vi "Initialize CAN.vi"(8 "error in (no error)":errorcluster, 11 "Parameters":T1={"Properties"={"Name"="", "CAN"={"Database File"=path "", "CAN Interface"=enum."CAN0", "Baud Rate"=0, "Diagnostic Protocol"=enum."GMLAN", "Transport Protocol"=enum."ISO TP - Normal Mode", "Transmit ID"=0, "Receive ID"=0, "Transmit Extension"=0, "Receive Extension"=0, "Receive UUDT ID"=0, "Enable Stream"=TRUE, "VW TP Channel ID"=0, "Security"={"Source DLL Path"=path "", "Security Level"=1, "Target DLL Path"=path ""}, "Fill Frame"=FALSE, "Fill Byte"=255, "Termination"=FALSE}, "FPGA Settings"={"RT Bitfile Path"=path "", "RIO Device"=0, "Enable"=FALSE}, "PIDs"=[], "PID Lookup"=variant, "CPIDs"=[], "CPID Lookup"=variant, "DIDs"=[], "DID Lookup"=variant, "DPIDs"=[], "DPID Lookup"=variant, "DTC descriptor"={"DTC Byte Length"=2, "Status Byte Length"=1, "Add Data Byte Length"=1, "Byte Order"=enum."Motorola"}}, "ChanRefs"={"ToVS.PIDs"={"Name"="", "Write to VS Engine FIFO"=refnum, "Pairs"={"Refs"=[], "Values"=[]}}, "ToVS.DIDs"={"Name"="", "Write to VS Engine FIFO"=refnum, "Pairs"={"Refs"=[], "Values"=[]}}, "ToVS.DTCs"={"Name"="", "Write to VS Engine FIFO"=refnum, "Pairs"={"Refs"=[], "Values"=[]}}, "ToVS.DTCCount"={"Name"="", "Write to VS Engine FIFO"=refnum, "Pairs"={"Refs"=[], "Values"=[]}}, "ToVS.Success"={"Name"="", "Write to VS Engine FIFO"=refnum, "Pairs"={"Refs"=[], "Values"=[]}}, "FromVS.CPIDs"={"Name"="", "Read from VS Engine FIFO"=refnum, "Pairs"={"Refs"=[], "Values"=[]}}, "Cmds"={"Name"="", "Write to VS Engine FIFO"=refnum, "Read from VS Engine FIFO"=refnum, "Pairs"={"Chan Refs"=[], "Prev. Values"=[]}}}} {"ChanRefs"."Cmds"."Pairs"."Chan Refs" format="%.0x"; "ChanRefs"."FromVS.CPIDs"."Pairs"."Refs"."Data Reference" format="%.0x"; "ChanRefs"."ToVS.Success"."Pairs"."Refs" format="%.0x"; "ChanRefs"."ToVS.DTCCount"."Pairs"."Refs" format="%.0x"; "ChanRefs"."ToVS.DTCs"."Pairs"."Refs" format="%.0x"; "ChanRefs"."ToVS.PIDs"."Pairs"."Refs" format="%.0x"; "ChanRefs"."ToVS.DIDs"."Pairs"."Refs" format="%.0x"; "Properties"."CPIDs"."Signals"."Byte Order" items=["Little Endian", "Big Endian"]; "Properties"."CPIDs"."Signals"."Data Type" items=["Signed", "Unsigned", "IEEE Float"]; "Properties"."DIDs"."Signals"."Byte Order" items=["Little Endian", "Big Endian"]; "Properties"."DIDs"."Signals"."Data Type" items=["Signed", "Unsigned", "IEEE Float"]; "Properties"."CAN"."Fill Byte" format="%.0x"; "Properties"."CAN"."VW TP Channel ID" format="%.0x"; "Properties"."CAN"."Receive UUDT ID" format="%.0x"; "Properties"."CAN"."Receive Extension" format="%.0x"; "Properties"."CAN"."Transmit Extension" format="%.0x"; "Properties"."CAN"."Receive ID" format="%.0x"; "Properties"."CAN"."Transmit ID" format="%.0x"; "Properties"."PIDs"."Signals"."Byte Order" items=["Little Endian", "Big Endian"]; "Properties"."PIDs"."Signals"."Data Type" items=["Signed", "Unsigned", "IEEE Float"]}) -> (0 "error out":errorcluster, 1 "ADCS Connection":T21, 2 "XNET References":T20, 3 "Parameters":T1={"Properties"={"Name"="", "CAN"={"Database File"=path "", "CAN Interface"=enum."CAN0", "Baud Rate"=0, "Diagnostic Protocol"=enum."GMLAN", "Transport Protocol"=enum."ISO TP - Normal Mode", "Transmit ID"=0, "Receive ID"=0, "Transmit Extension"=0, "Receive Extension"=0, "Receive UUDT ID"=0, "Enable Stream"=TRUE, "VW TP Channel ID"=0, "Security"={"Source DLL Path"=path "", "Security Level"=1, "Target DLL Path"=path ""}, "Fill Frame"=FALSE, "Fill Byte"=255, "Termination"=FALSE}, "FPGA Settings"={"RT Bitfile Path"=path "", "RIO Device"=0, "Enable"=FALSE}, "PIDs"=[], "PID Lookup"=variant, "CPIDs"=[], "CPID Lookup"=variant, "DIDs"=[], "DID Lookup"=variant, "DPIDs"=[], "DPID Lookup"=variant, "DTC descriptor"={"DTC Byte Length"=2, "Status Byte Length"=1, "Add Data Byte Length"=1, "Byte Order"=enum."Motorola"}}, "ChanRefs"={"ToVS.PIDs"={"Name"="", "Write to VS Engine FIFO"=refnum, "Pairs"={"Refs"=[], "Values"=[]}}, "ToVS.DIDs"={"Name"="", "Write to VS Engine FIFO"=refnum, "Pairs"={"Refs"=[], "Values"=[]}}, "ToVS.DTCs"={"Name"="", "Write to VS Engine FIFO"=refnum, "Pairs"={"Refs"=[], "Values"=[]}}, "ToVS.DTCCount"={"Name"="", "Write to VS Engine FIFO"=refnum, "Pairs"={"Refs"=[], "Values"=[]}}, "ToVS.Success"={"Name"="", "Write to VS Engine FIFO"=refnum, "Pairs"={"Refs"=[], "Values"=[]}}, "FromVS.CPIDs"={"Name"="", "Read from VS Engine FIFO"=refnum, "Pairs"={"Refs"=[], "Values"=[]}}, "Cmds"={"Name"="", "Write to VS Engine FIFO"=refnum, "Read from VS Engine FIFO"=refnum, "Pairs"={"Chan Refs"=[], "Prev. Values"=[]}}}} {"ChanRefs"."Cmds"."Pairs"."Chan Refs" format="%.0x"; "ChanRefs"."FromVS.CPIDs"."Pairs"."Refs"."Data Reference" format="%.0x"; "ChanRefs"."ToVS.Success"."Pairs"."Refs" format="%.0x"; "ChanRefs"."ToVS.DTCCount"."Pairs"."Refs" format="%.0x"; "ChanRefs"."ToVS.DTCs"."Pairs"."Refs" format="%.0x"; "ChanRefs"."ToVS.PIDs"."Pairs"."Refs" format="%.0x"; "ChanRefs"."ToVS.DIDs"."Pairs"."Refs" format="%.0x"; "Properties"."CPIDs"."Signals"."Byte Order" items=["Little Endian", "Big Endian"]; "Properties"."CPIDs"."Signals"."Data Type" items=["Signed", "Unsigned", "IEEE Float"]; "Properties"."DIDs"."Signals"."Byte Order" items=["Little Endian", "Big Endian"]; "Properties"."DIDs"."Signals"."Data Type" items=["Signed", "Unsigned", "IEEE Float"]; "Properties"."CAN"."Fill Byte" format="%.0x"; "Properties"."CAN"."VW TP Channel ID" format="%.0x"; "Properties"."CAN"."Receive UUDT ID" format="%.0x"; "Properties"."CAN"."Receive Extension" format="%.0x"; "Properties"."CAN"."Transmit Extension" format="%.0x"; "Properties"."CAN"."Receive ID" format="%.0x"; "Properties"."CAN"."Transmit ID" format="%.0x"; "Properties"."PIDs"."Signals"."Byte Order" items=["Little Endian", "Big Endian"]; "Properties"."PIDs"."Signals"."Data Type" items=["Signed", "Unsigned", "IEEE Float"]})   [LabVIEW 2015, in "Diagnostics Addon Engine.lvlib"]
uses:
  Diagnostics Addon Engine.lvlib
  Main Configuration.ctl
  Shared/Section Properties.ctl
  Shared/CAN Configuration.ctl
  Shared/CAN Interface.ctl
  Shared/Diagnostic Protocols.ctl
  Shared/Transport Protocols.ctl
  Shared/Security.ctl
  Shared/FPGA Bitfile Settings.ctl
  Shared/Frame Parameters.ctl
  Shared/Signal Parameters.ctl
  Shared/DPID Parameters.ctl
  Shared/DPID Periodic Rate.ctl
  <vilib>/Automotive Diagnostic Command Set/Diagnostic Protocols.llb/DTC Descriptor.ctl
  VS Data Channels.ctl
  Inline Async API/Controls/Write To VS Engine.ctl
  <vilib>/NI Veristand/Custom Device API/Data Reference.ctl
  Inline Async API/Controls/Read From VS Engine.ctl
  <vilib>/NI Veristand/Custom Device API/Block Data Reference.ctl
  Inline Async API/Controls/ReadWrite Data.ctl
  <vilib>/Automotive Diagnostic Command Set/Diagnostic Transport.llb/Diag Reference.ctl
  <vilib>/Automotive Diagnostic Command Set/Diagnostic Transport.llb/Transport Protocol Selector.ctl
  <vilib>/Automotive Diagnostic Command Set/Diagnostic Transport.llb/Diag CAN Frame Log.ctl
  XNET References.ctl
  <vilib>/Automotive Diagnostic Command Set/Diagnostic Transport.llb/Property ID.ctl
  DIDPID Selector.ctl
  <vilib>/Automotive Diagnostic Command Set/Diagnostic Transport.llb/VWTP Application Type.ctl
  <vilib>/Automotive Diagnostic Command Set/Diagnostic Transport.llb/DoIP OpenType.ctl
  <vilib>/xnet/xnet.llb/XNET Create Session (Frame Input Queued).vi
  <vilib>/addons/Automotive Diagnostic Command Set/NI_Automotive Diagnostic Command Set.lvlib
  <vilib>/NI Veristand/Custom Device Tools/Custom Device Utility Library/Custom Device Utility Library.lvlib
  Shared/Diagnostics Addon Shared.lvlib
  <vilib>/NI Veristand/Custom Device API/Custom Device API.lvlib
  Inline Async API/Inline Async API.lvlib
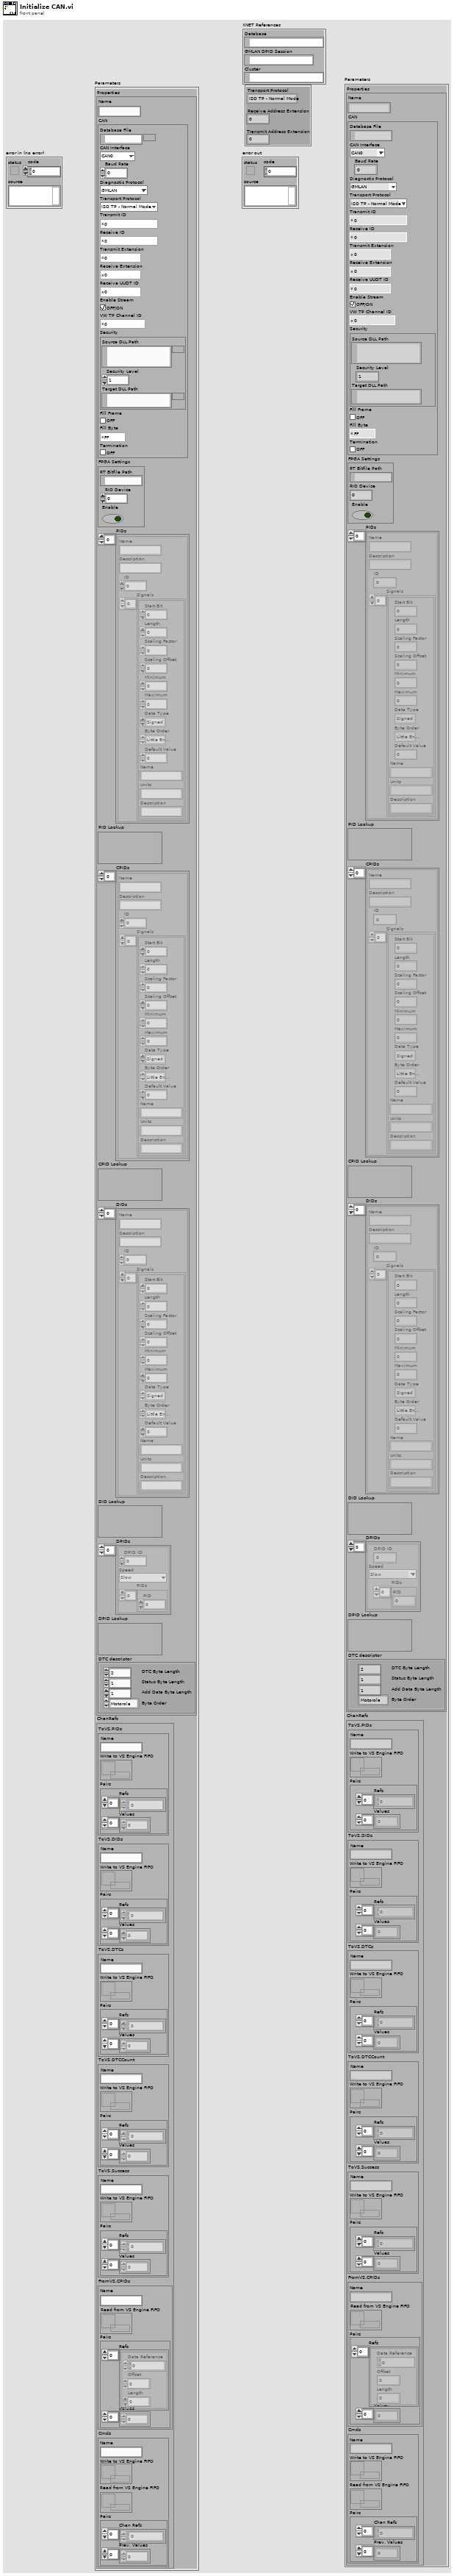
[diagram p1: front panel]
types:
  T1 = typedef "Diagnostics Addon Engine.lvlib/Main Configuration.ctl" = cluster{"Properties":T2, "ChanRefs":T14}
  T2 = typedef "Diagnostics Addon Shared.lvlib/Section Properties.ctl" = cluster{"Name":string, "CAN":T3, "FPGA Settings":T8, "PIDs":T9[], "PID Lookup":variant, "CPIDs":T9[], "CPID Lookup":variant, "DIDs":T9[], "DID Lookup":variant, "DPIDs":T11[], "DPID Lookup":variant, "DTC descriptor":T13}
  T3 = typedef "Diagnostics Addon Shared.lvlib/CAN Configuration.ctl" = cluster{"Database File":path, "CAN Interface":T4, "Baud Rate":u32, "Diagnostic Protocol":T5, "Transport Protocol":T6, "Transmit ID":u32, "Receive ID":u32, "Transmit Extension":u8, "Receive Extension":u8, "Receive UUDT ID":u32, "Enable Stream":bool, "VW TP Channel ID":u32, "Security":T7, "Fill Frame":bool, "Fill Byte":u8, "Termination":bool}
  T4 = typedef "Diagnostics Addon Shared.lvlib/CAN Interface.ctl" = enum16{"CAN0", "CAN1", "CAN2", "CAN3", "CAN4", "CAN5", "CAN6", "CAN7", "CAN8", "CAN9", "CAN10", "CAN11", "CAN12", "CAN13", "CAN14", "CAN15", "CAN16", "CAN17", "CAN18", "CAN19", "CAN20", "CAN21", "CAN22", "CAN23", "CAN24", "CAN25", "CAN26", "CAN27", "CAN28", "CAN29", "CAN30", "CAN31", "CAN32", "CAN33", "CAN34", "CAN35", "CAN36", "CAN37", "CAN38", "CAN39", "CAN40", "CAN41", "CAN42", "CAN43", "CAN44", "CAN45", "CAN46", "CAN47", "CAN48", "CAN49", "CAN50", "CAN51", "CAN52", "CAN53", "CAN54", "CAN55", "CAN56", "CAN57", "CAN58", "CAN59", "CAN60", "CAN61", "CAN62", "CAN63", "CAN 256 (Virtual)", "CAN 257 (Virtual)"}
  T5 = typedef "Diagnostics Addon Shared.lvlib/Diagnostic Protocols.ctl" = enum16{"GMLAN", "KWP-2000", "UDS"}
  T6 = typedef "Diagnostics Addon Shared.lvlib/Transport Protocols.ctl" = enum16{"ISO TP - Normal Mode", "ISO TP - Mixed Mode", "VW TP 2.0", "Diagnostics on IP"}
  T7 = typedef "Diagnostics Addon Shared.lvlib/Security.ctl" = cluster{"Source DLL Path":path, "Security Level":u8, "Target DLL Path":path}
  T8 = typedef "Diagnostics Addon Shared.lvlib/FPGA Bitfile Settings.ctl" = cluster{"RT Bitfile Path":path, "RIO Device":u16, "Enable":bool}
  T9 = typedef "Diagnostics Addon Shared.lvlib/Frame Parameters.ctl" = cluster{"Name":string, "Description":string, "ID":u16, "Signals":T10[]}
  T10 = typedef "Diagnostics Addon Shared.lvlib/Signal Parameters.ctl" = cluster{"Start Bit":u8, "Length":u8, "Scaling Factor":dbl, "Scaling Offset":dbl, "Minimum":dbl, "Maximum":dbl, "Data Type":u32, "Byte Order":u32, "Default Value":dbl, "Name":string, "Units":string, "Description":string}
  T11 = typedef "Diagnostics Addon Shared.lvlib/DPID Parameters.ctl" = cluster{"DPID ID":u8, "Speed":T12, "PIDs":u16[]}
  T12 = typedef "Diagnostics Addon Shared.lvlib/DPID Periodic Rate.ctl" = enum16{"Slow", "Medium", "Fast"}
  T13 = typedef "Diagnostics Addon Shared.lvlib/DTC Descriptor.ctl" = cluster{"DTC Byte Length":i32, "Status Byte Length":i32, "Add Data Byte Length":i32, "Byte Order":enum16{"Motorola", "Intel"}}
  T14 = typedef "Diagnostics Addon Engine.lvlib/VS Data Channels.ctl" = cluster{"ToVS.PIDs":T15, "ToVS.DIDs":T15, "ToVS.DTCs":T15, "ToVS.DTCCount":T15, "ToVS.Success":T15, "FromVS.CPIDs":T17, "Cmds":T19}
  T15 = typedef "Diagnostics Addon Engine.lvlib/Inline Async API.lvlib/Write To VS Engine.ctl" = cluster{"Name":string, "Write to VS Engine FIFO":refnum<k33>, "Pairs":cluster{"Refs":T16[], "Values":dbl[]}}
  T16 = typedef "Custom Device API.lvlib/Data Reference.ctl" = i32
  T17 = typedef "Diagnostics Addon Engine.lvlib/Inline Async API.lvlib/Read From VS Engine.ctl" = cluster{"Name":string, "Read from VS Engine FIFO":refnum<k33>, "Pairs":cluster{"Refs":T18[], "Values":dbl[]}}
  T18 = typedef "Custom Device API.lvlib/Block Data Reference.ctl" = cluster{"Data Reference":T16, "Offset":u64, "Length":u64}
  T19 = typedef "Diagnostics Addon Engine.lvlib/Inline Async API.lvlib/ReadWrite Data.ctl" = cluster{"Name":string, "Write to VS Engine FIFO":refnum<k33>, "Read from VS Engine FIFO":refnum<k33>, "Pairs":cluster{"Chan Refs":T16[], "Prev. Values":dbl[]}}
  T20 = typedef "Diagnostics Addon Engine.lvlib/XNET References.ctl" = cluster{"Database":refnum<k21>, "GMLAN DPID Session":refnum<k21>, "Cluster":refnum<k21>}
  T21 = typedef "NI_Automotive Diagnostic Command Set.lvlib/Diag Reference.ctl" = cluster{"Diag CAN Handle":u32, "Transport Protocol":T22, "Receive Address Extension":u8, "Transmit Address Extension":u8, "Receive CAN Id":u32, "Transmit CAN Id":u32, "Diag CAN Queue":refnum<queue>, "Log Frames ?":bool, "My TP Address":u8, "Other TP Address":u8, "T1":u16, "T2":u16, "T3":u16, "T4":u16, "Tx SN":u8, "Block Size":u8, "Rx SN":u8, "VW TP Initialized?":bool, "Tx block no":u8, "baud rate":u32, "Interface":string, "Channel Diag CAN Handle":u32, "UDP Connection ID":refnum<k16>, "TCP Connection ID":refnum<k5>, "Target IP Addr":u32, "Source Address":u16, "Target Address":u16, "Send Header NACK?":bool, "DLL Handle":u32, "NAD":u8, "Time Stamp read first":dbl, "Time Stamp read last":dbl, "Time Stamp write first":dbl, "Time Stamp write last":dbl, "Time Stamp write":dbl, "Time Stamp read":dbl}
  T22 = typedef "NI_Automotive Diagnostic Command Set.lvlib/Transport Protocol Selector.ctl" = enum16{"ISO TP - Normal Mode", "ISO TP - Mixed Mode", "VW TP 2.0", "Diagnostics on IP", "ISO TP LIN"}
  T23 = typedef "NI_Automotive Diagnostic Command Set.lvlib/Property ID.ctl" = enum16{"Timeout Diag Command", "Timeout FC (Bs)", "Timeout CF (Cr)", "Receive Block Size (BS)", "Wait Time CF (STmin)", "Max Wait Frames (N_WFTmax)", "Wait Frames to Send (N_WAIT)", "Time between Waits (T_W)", "Fill CAN Frames", "Fill Byte", "Invalid Response as Error", "Max RspPending Count", "VWTP Command Timeout", "STmin", "P2min", "Termination"}
  T24 = typedef "Diagnostics Addon Engine.lvlib/DIDPID Selector.ctl" = enum16{"DID", "PID", "CPID"}
  T25 = typedef "NI_Automotive Diagnostic Command Set.lvlib/VWTP Application Type.ctl" = u8
  T26 = typedef "NI_Automotive Diagnostic Command Set.lvlib/DoIP OpenType.ctl" = u16
  T27 = typedef "NI_Automotive Diagnostic Command Set.lvlib/DoIP Vehicle ID Cluster.ctl" = cluster{"VIN":string, "Source Address":u16, "EID":u8[], "GID":u8[], "IP Address":string}
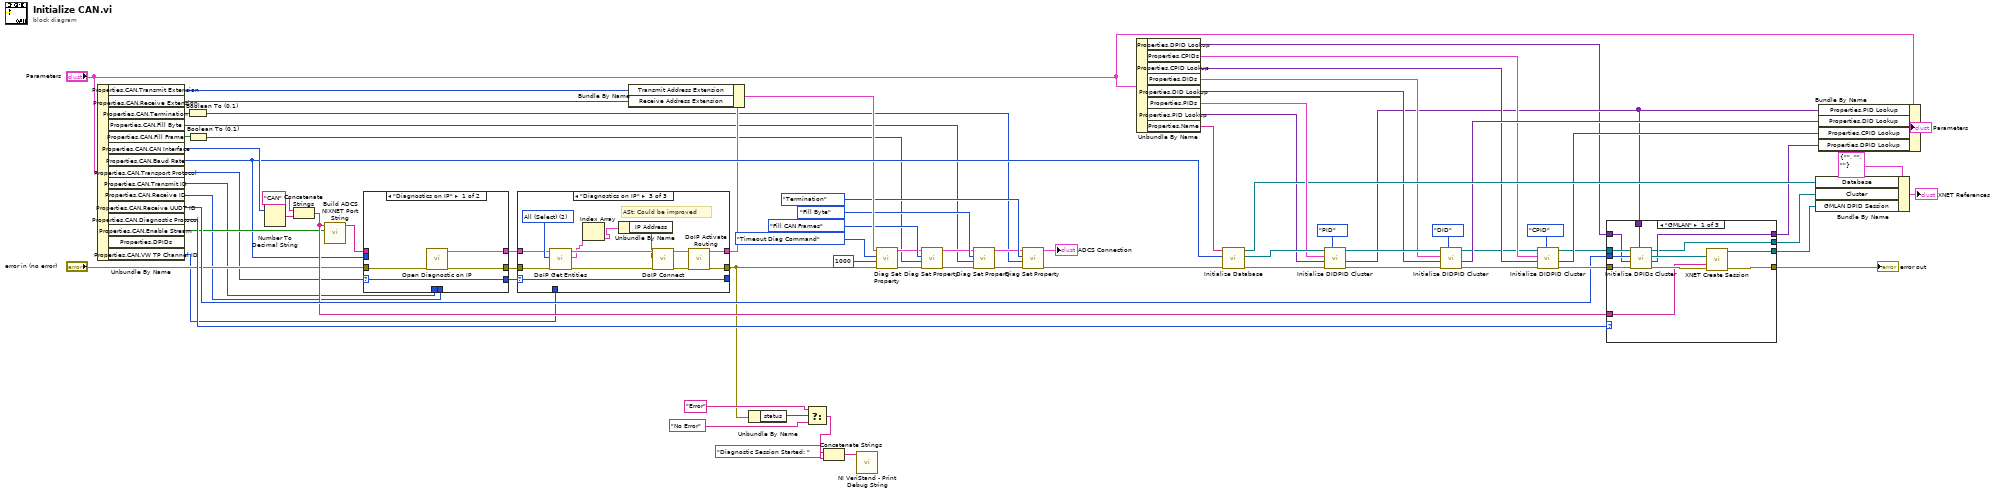
[diagram p0: block diagram]
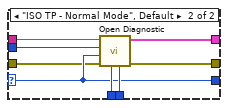
[diagram p2: hidden frame]
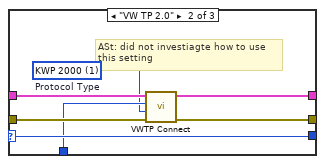
[diagram p4: hidden frame]
diagram:
  n1 = Unbundle By Name("Parameters") -> ("Properties.CAN.Transmit Extension"=w74:u8, "Properties.CAN.Receive Extension"=w73:u8, "Properties.CAN.Termination"=w3:bool, "Properties.CAN.Fill Byte"=w5:u8, "Properties.CAN.Fill Frame"=w4:bool, "Properties.CAN.CAN Interface"=w77:T4, "Properties.CAN.Baud Rate"=w25:u32, "Properties.CAN.Transport Protocol"=w28:T6, "Properties.CAN.Transmit ID"=w24:u32, "Properties.CAN.Receive ID"=w23:u32, "Properties.CAN.Receive UUDT ID"=w44:u32, "Properties.CAN.Diagnostic Protocol"=w43:T5, "Properties.CAN.Enable Stream"=w37:bool, "Properties.CAN.VW TP Channel ID"=w18:u32)  [unwired: 1 out]
  n2 = Boolean To (0,1)(Boolean=w3) -> (0, 1=w2:i16)
  n3 = Boolean To (0,1)(Boolean=w4) -> (0, 1=w1:i16)
  n4 = Number To Decimal String(number=w77) -> (decimal integer string=w76:string)  [unwired: 1 in]
  n5 = Concatenate Strings("CAN" ("string"), w76) -> (w38:string)
  n6 = call "Build ADCS NIXNET Port String.vi"("Enable Stream"=w37, "CAN port"=w38) -> ("CAN port out"=w26:string)  [unwired: 9 in]
  n7 = case shown="\"Diagnostics on IP\"" w28 {
    selector: w28 -> [w81 w83]
    tunnel: w24 -> [_ w89]
    tunnel: w25 -> [_ w88]
    tunnel: w23 -> [_ w87]
    tunnel: [w79 w86] -> w22
    tunnel: [w80 w85] -> w20
    tunnel: w26 -> [_ w84]
    tunnel: [w81 w83] -> w27
    tunnel: "error in (no error)" -> [w78 w82]
    frame "Diagnostics on IP" {
      n8 = call <vilib>:"Open Diagnostic on IP.vi"("error in (no error)"=w78) -> ("error out"=w80:errorcluster, "Diag reference out"=w79:T21)  [unwired: 1 in, 8 out]
    }
    frame "ISO TP - Normal Mode", Default {
      n9 = call <vilib>:"Open Diagnostic.vi"("Receive ID"=w87, "Transmit ID"=w89, "error in (no error)"=w82, "Transport Protocol"=w83, "Baud Rate"=w88, "CAN Interface"=w84) -> ("error out"=w85:errorcluster, "diag ref out"=w86:T21)  [unwired: 4 out]
    }
  }
  n10 = case shown="\"Diagnostics on IP\"" w27 {
    selector: w27 -> [w92 w97 w102]
    tunnel: [w91 w99 w105] -> w21
    tunnel: [w90 w98 w103] -> w19
    tunnel: [w92 w97 w102] -> _
    tunnel: w22 -> [w91 w96 w101]
    tunnel: w20 -> [w90 w95 w100]
    tunnel: w18 -> [_ w94 _]
    frame "ISO TP - Normal Mode", Default {
    }
    frame "VW TP 2.0" {
      w93 = T25 1 items=["KWP 2000"=1, "KS Type 010C"=2, "Infotainment communication"=16, "Application protocol"=32, "WFS/WIV"=33]  # Protocol Type
      # "ASt: did not investiagte how to use\nthis setting"
      n11 = call <vilib>:"VWTP Connect.vi"("error in"=w95, "application type"=w93, "channel ID"=w94, "diag ref in"=w96) -> ("error out"=w98:errorcluster, "diag ref out"=w99:T21)  [unwired: 6 out]
    }
    frame "Diagnostics on IP" {
      w112 = T26 2 items=["VIN", "EID", "All (Select)"] ("DoIP Open Type")
      # "ASt: Could be improved"
      n12 = call <vilib>:"DoIP Get Entities.vi"("error in (no error)"=w100, "DoIP Open Type"=w112, "Diag reference in"=w101) -> ("error out"=w109:errorcluster, "DoIP entities"=w108:T27[], "Diag reference out"=w110:T21)  [unwired: 1 in, 5 out]
      n13 = Index Array(array=w108) -> (element=w107:T27)  [unwired: 1 in]
      n14 = Unbundle By Name(w107) -> ("IP Address"=w106:string)
      n15 = call <vilib>:"DoIP Connect.vi"("error in (no error)"=w109, "address"=w106, "Diag Reference in"=w110) -> ("error out"=w104:errorcluster, "Diag reference out"=w111:T21)  [unwired: 2 in, 5 out]
      n16 = call <vilib>:"DoIP Activate Routing.vi"("error in (no error)"=w104, "Diag reference in"=w111) -> ("error out"=w103:errorcluster, "Diag reference out"=w105:T21)  [unwired: 2 in, 6 out]
    }
  }
  n17 = Bundle By Name(cluster=w21, "Transmit Address Extension"=w74, "Receive Address Extension"=w73) -> (w17:T21)
  n18 = Unbundle By Name(w19) -> ("status"=w34:bool)
  n19 = Select(t="Error" ("string"), s=w34, f="No Error" ("string")) -> (s? t:f=w31:string)
  n20 = Concatenate Strings("Diagnostic Session Started: " ("string"), w31) -> (w30:string)
  n21 = call <vilib>:"NI VeriStand - Print Debug String.vi"("Message"=w30) -> ()  [unwired: 10 in, 1 out]
  n22 = call <vilib>:"Diag Set Property.vi"("error in (no error)"=w19, "property value"=u32 1000, "property ID"=Property_ID."Timeout Diag Command", "diag ref in"=w17) -> ("error out"=w14:errorcluster, "diag ref out"=w9:T21)  [unwired: 6 in]
  n23 = call <vilib>:"Diag Set Property.vi"("error in (no error)"=w14, "property value"=w1, "property ID"=Property_ID."Fill CAN Frames", "diag ref in"=w9) -> ("error out"=w16:errorcluster, "diag ref out"=w8:T21)  [unwired: 6 in]
  n24 = call <vilib>:"Diag Set Property.vi"("error in (no error)"=w16, "property value"=w5, "property ID"=Property_ID."Fill Byte", "diag ref in"=w8) -> ("error out"=w15:errorcluster, "diag ref out"=w7:T21)  [unwired: 6 in]
  n25 = call <vilib>:"Diag Set Property.vi"("error in (no error)"=w15, "property value"=w2, "property ID"=Property_ID."Termination", "diag ref in"=w7) -> ("error out"=w13:errorcluster, "diag ref out"=→"ADCS Connection":T21)  [unwired: 6 in]
  n26 = Unbundle By Name("Parameters") -> ("Properties.DPID Lookup"=w40:variant, "Properties.CPIDs"=w50:T9[], "Properties.CPID Lookup"=w51:variant, "Properties.DIDs"=w58:T9[], "Properties.DID Lookup"=w55:variant, "Properties.PIDs"=w60:T9[], "Properties.PID Lookup"=w56:variant, "Properties.Name"=w57:string)
  n27 = call "Initialize Database.vi"("error in (no error)"=w13, "Baud Rate"=w25, "Addon Name"=w57) -> ("error out"=w67:errorcluster, "Cluster"=w65:refnum<k21>, "XNET Database"=w59:refnum<k21>)  [unwired: 6 in]
  n28 = call "Initialize DIDPID Cluster.vi"("DID/PID Selector"=DIDPID_Selector."PID", "error in"=w67, "Lookup"=w56, "DIDs/PIDs"=w60, "Cluster In"=w65) -> ("error out"=w66:errorcluster, "DID Lookup Out"=w41:variant, "Cluster Out"=w62:refnum<k21>)  [unwired: 4 in]
  n29 = call "Initialize DIDPID Cluster.vi"("DID/PID Selector"=DIDPID_Selector."DID", "error in"=w66, "Lookup"=w55, "DIDs/PIDs"=w58, "Cluster In"=w62) -> ("error out"=w52:errorcluster, "DID Lookup Out"=w54:variant, "Cluster Out"=w49:refnum<k21>)  [unwired: 4 in]
  n30 = call "Initialize DIDPID Cluster.vi"("DID/PID Selector"=DIDPID_Selector."CPID", "error in"=w52, "Lookup"=w51, "DIDs/PIDs"=w50, "Cluster In"=w49) -> ("error out"=w47:errorcluster, "DID Lookup Out"=w48:variant, "Cluster Out"=w45:refnum<k21>)  [unwired: 4 in]
  n31 = case shown="\"GMLAN\"" w43 {
    tunnel: w47 -> [w122 w127 w130]
    tunnel: [w114 w127 w130] -> w46
    tunnel: w38 -> [w121 _ _]
    tunnel: w45 -> [w120 w125 w128]
    tunnel: w44 -> [w119 _ _]
    tunnel: [w118 _ _] -> w42
    tunnel: w41 -> [w117 _ _]
    tunnel: w40 -> [w116 w126 w129]
    tunnel: [w115 w126 w129] -> w39
    tunnel: [w113 w125 w128] -> w36
    frame "GMLAN" {
      n32 = call "Initialize DPIDs Cluster.vi"("PID Lookup"=w117, "error in"=w122, "DPID Lookup"=w116, "UUDT Receive ID"=w119, "cluster in"=w120) -> ("error out"=w123:errorcluster, "DPID Lookup Out"=w115:variant, "GMLAN DPID Session"=w124:refnum<k21>, "Cluster Out"=w113:refnum<k21>)  [unwired: 3 in]
      n33 = call-poly <vilib>:"XNET Create Session.vi"("frame"=w124, "interface"=w121, "error in (no error)"=w123) -> ("session out"=w118:refnum<k21>, "error out"=w114:errorcluster)  [unwired: 11 out]
    }
    frame "KWP-2000" {
    }
    frame "UDS" {
    }
  }
  "error out" <- w46
  n34 = Bundle By Name(cluster=T20 {"Database"="", "GMLAN DPID Session"="", "Cluster"=""}, "Database"=w59, "Cluster"=w36, "GMLAN DPID Session"=w42) -> (→"XNET References":T20)
  n35 = Bundle By Name(cluster="Parameters", "Properties.PID Lookup"=w41, "Properties.DID Lookup"=w54, "Properties.CPID Lookup"=w48, "Properties.DPID Lookup"=w39) -> (→"Parameters":T1)
